vi "Create Property Node.vi"   [LabVIEW 2012, in "Scripting Tools.lvlib"]
uses:
  Scripting Tools.lvlib
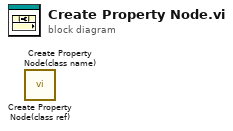
[diagram p0: block diagram]
diagram:
  n1 = call "Create Property Node(class ref).vi"() -> ()  [unwired: 11 in, 5 out]
  n2 = call "Create Property Node(class name).vi"() -> ()  [unwired: 11 in, 5 out]
